vi "check csi fifo load.vi"(10 "csi num":u32, 11 "Refnum in":T1) -> (2 "Boolean":bool, 3 "CSI Remaining":u32)   [LabVIEW 2020]
uses:
  Host/SubVIs/Streaming Xvcr FPGA Ref.ctl
  <vilib>/Utility/error.llb/Error Cluster From Error Code.vi
  <vilib>/rvi/errors/niLvFpgaAdjustHostInterfaceError.vi
  <vilib>/rvi/interface/nirviMethod/nirviMethod.xnode
  <vilib>/FPGAPlugInAG/Dynamic/niLvFpga_ReadFifo_Dynamic.vi
  <vilib>/rvi/errors/niLvFpgaMergeErrorWithErrorCode.vi
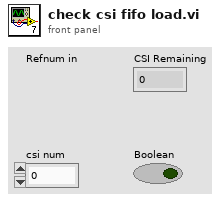
[diagram p1: front panel]
types:
  T1 = typedef "Streaming Xvcr FPGA Ref.ctl" = refnum<k20>
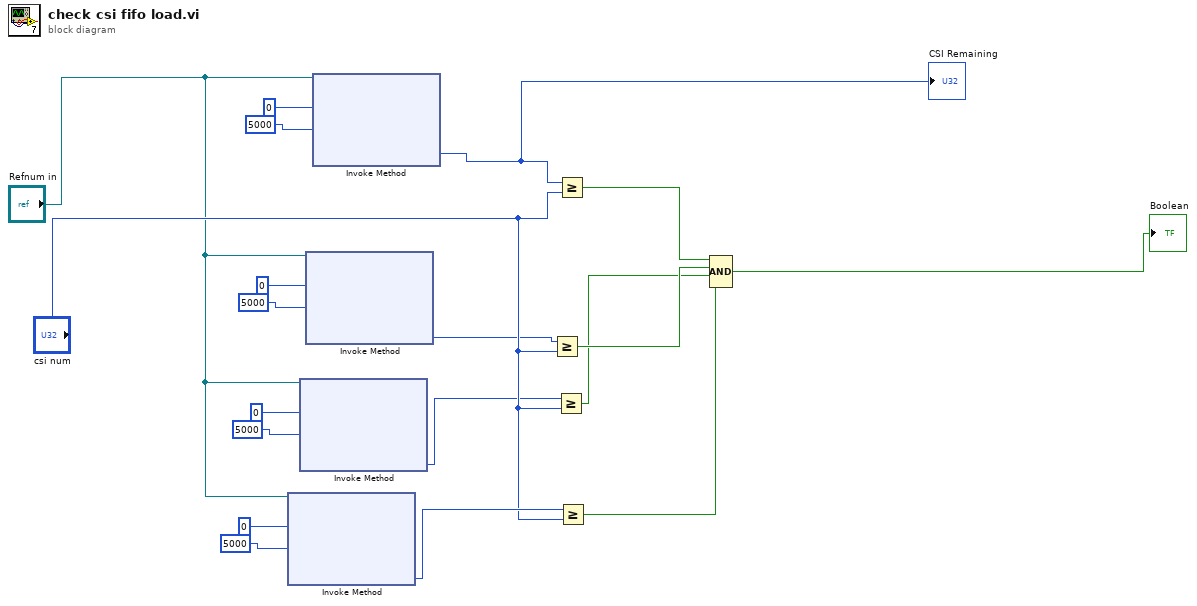
[diagram p0: block diagram]
diagram:
  n1 = xnode "Invoke Method"("FPGA VI Reference In"="Refnum in", "Number of Elements"=u32 0, "Timeout (ms)"=5000) -> ("Elements Remaining"=w10:u32)  [unwired: 1 in, 3 out]
  n2 = xnode "Invoke Method"("FPGA VI Reference In"="Refnum in", "Number of Elements"=u32 0, "Timeout (ms)"=5000) -> ("Elements Remaining"=w7:u32)  [unwired: 1 in, 3 out]
  n3 = xnode "Invoke Method"("FPGA VI Reference In"="Refnum in", "Number of Elements"=u32 0, "Timeout (ms)"=5000) -> ("Elements Remaining"=w8:u32)  [unwired: 1 in, 3 out]
  n4 = xnode "Invoke Method"("FPGA VI Reference In"="Refnum in", "Number of Elements"=u32 0, "Timeout (ms)"=5000) -> ("Elements Remaining"=w17:u32)  [unwired: 1 in, 3 out]
  "CSI Remaining" <- w17
  n5 = Greater Or Equal?(x=w8, y="csi num") -> (x >= y?=w5:bool)
  n6 = Greater Or Equal?(x=w7, y="csi num") -> (x >= y?=w4:bool)
  n7 = Greater Or Equal?(x=w17, y="csi num") -> (x >= y?=w6:bool)
  n8 = Greater Or Equal?(x=w10, y="csi num") -> (x >= y?=w3:bool)
  n9 = Compound Arithmetic op=AND(w6, w5, w4, w3) -> (→"Boolean":bool)
